vi "PH_Sequencer_Watch.panel.vi"() -> ()   [LabVIEW 2014, in "PH_Sequencer_Watch.lvlib"]
uses:
  PH_Sequencer_Watch.lvlib
  PH_Beamline_Chief/PH_Beamline_Chief.Section.ctl
  PH_Basics/PH_SystemInformation/PH_SystemInformation.GUI Refs.ctl
  PH_BeamlineInformation/PH_BeamlineInformation.Powermeter.ctl
  PH_BeamlineInformation/PH_BeamlineInformation.Efficiency.ctl
  PH_Basics/PH_PP_Common/PH_PP_Common.PUs.ctl
  PH_Sequencer_Watch.Head Information.ctl
  PH_BeamlineInformation/PH_BeamlineInformation.GUI Ref.ctl
  PH_Basics/PH_Common/PH_Common.lvlib
  PH_Beamline_Chief/PH_Beamline_Chief.lvlib
  PH_BeamlineInformation/PH_BeamlineInformation.lvlib
  PH_Basics/PH_PP_Common/PH_PP_Common.lvlib
  PH_Basics/PH_SystemInformation/PH_SystemInformation.lvlib
  PH_Basics/PH_Class/PH_Class.lvlib
panel:
  out "PA 45 DP Voltage":cluster{dbl, dbl}(slide)={99999.0, 0.0} scale=0.0..20.0
  out "PPPA 45mm DP":bool caption="45 DP"
  out "PA 45 Voltage":cluster{dbl, dbl}(slide)={99999.0, 0.0} scale=0.0..20.0
  out "PPPA_45mm_MAIN_PU":bool caption="45"
  out "PA 19-2 Voltage":cluster{dbl, dbl}(slide)={99999.0, 0.0} scale=0.0..20.0
  out "PPPA_19mm_2_PU":bool caption="19-2"
  out "PA 19-1 Voltage":cluster{dbl, dbl}(slide)={99999.0, 0.0} scale=0.0..20.0
  out "PPPA_19mm_1_PU":bool caption="State PU"
  out "Z6_COS_Powermeter_CurrentValue":dbl=-1.0 caption="mJ"
  out "Z6_IR_Powermeter_CurrentValue":dbl=-1.0 caption="J"
  out "Z6_green_Powermeter_CurrentValue":dbl=-1.0 caption="J"
  out "PHELIX_Beamline_MA_LB_BL_Status 2":u32(colorbox)
  out "Experiment_VacuumControl_Experiment":bool caption="V"
  out "PA-Backreflection-Meas":bool caption="B"
  out "fs_Synchrolock_Watch":bool caption="S"
  in  "T2-Unit-Dummy":string caption="s"
  out "PHELIX_Timing_T2":i16 caption="T2"
  out "PHELIX_Beamline_PA_before_Bypass_BL_Status":u32(colorbox)
  out "PHELIX_Beamline_PA_BL_Status":u32(colorbox)
  out "PHELIX_Beamline_LB_TB2_BL_Status":u32(colorbox)
  out "PHELIX_Beamline_Z6_BL_Status":u32(colorbox)
  out "PHELIX_Beamline_LL_BL_Status":u32(colorbox)
  out "PHELIX_Beamline_MA_Exit_BL_Status":u32(colorbox)
  out "PHELIX_Beamline_PA_Exit_BL_Status":u32(colorbox)
  out "PHELIX_Beamline_PA_Input_BL_Status":u32(colorbox)
  out "PHELIX_Beamline_PA_UnDelay_BL_Status":u32(colorbox)
  out "PHELIX_Beamline_fs_YLF_BL_Status":u32(colorbox)
  out "PHELIX_Beamline_YLF_BL_Status 2":u32(colorbox)
  out "PHELIX_Beamline_ns_BL_Status 2":u32(colorbox)
  out "PHELIX_Beamline_PA_Bypass_BL_Status 3":u32(colorbox)
  out "PHELIX_Beamline_PA_Bypass_BL_Status 2":u32(colorbox)
  out "PHELIX_Beamline_PA_Bypass_BL_Status 1":u32(colorbox)
  out "PHELIX_Beamline_PA_Delay_BL_Status 3":u32(colorbox)
  out "PHELIX_Beamline_PA_Delay_BL_Status 1":u32(colorbox)
  out "PHELIX_Beamline_PA_Delay_BL_Status 2":u32(colorbox)
  out "PHELIX_Beamline_MA_Z6_BL_Status":u32(colorbox)
  out "PA_Exit_Powermeter_CurrentValue":dbl=-1.0 caption="J"
  out "MAS_Powermeter_CurrentValue":dbl=-1.0 caption="J"
  out "PHELIX_Beamline_MA_LB_BL_Status 1":u32(colorbox)
  out "PHELIX_Beamline_MA_LB_BL_Status":u32(colorbox)
  out "PHELIX_Beamline_YLF_BL_Status 1":u32(colorbox)
  out "PHELIX_Beamline_fs_BL_Status":u32(colorbox)
  out "PHELIX_Beamline_ns_BL_Status 1":u32(colorbox)
  out "PHELIX_Beamline_PA_LL_BL_Status 2":u32(colorbox)
  out "PHELIX_Beamline_PA_LL_BL_Status 1":u32(colorbox)
  out "PHELIX_Beamline_PA_MA_BL_Status":u32(colorbox)
  out "Countdown_Remaining_Time":string caption="ing_Time"
  out "MA PU FR Voltage":cluster{dbl, dbl}(slide)={99999.0, 0.0} scale=0.0..20.0
  out "PPMA_FR":bool caption="State PU"
  out "MA PU 5 Voltage":cluster{dbl, dbl}(slide)={99999.0, 0.0} scale=0.0..20.0
  out "PPMA_PU5":bool caption="State PU"
  out "MA PU 4 Voltage":cluster{dbl, dbl}(slide)={99999.0, 0.0} scale=0.0..20.0
  out "PPMA_PU4":bool caption="State PU"
  out "MA PU 3 Voltage":cluster{dbl, dbl}(slide)={99999.0, 0.0} scale=0.0..20.0
  out "PPMA_PU3":bool caption="State PU"
  out "MA PU 2 Voltage":cluster{dbl, dbl}(slide)={99999.0, 0.0} scale=0.0..20.0
  out "PPMA_PU2":bool caption="State PU"
  out "MA PU 1 Voltage":cluster{dbl, dbl}(slide)={99999.0, 0.0} scale=0.0..20.0
  out "PPMA_PU1":bool caption="State PU"
  out "PHELIX_PSDB-Controller_Shot-ID":i32 caption="Shot ID"
  out "PHELIX_Sequencer_1":string="no info" caption="Sequencer State"
  out "PHELIX_Timing_Mode":enum32{"10 Hz", "0.5 Hz", "Shot"}(radio) caption="Modeselector"
  in  "Delete":bool
  out "PIL_Exp4_ShutterDisabled":u32(colorbox) caption="Z6 enabled"
  out "PIL_Exp1_ShutterDisabled":u32(colorbox) caption="Exp 1 enabled"
  out "PIL_Exp2_ShutterDisabled":u32(colorbox) caption="Exp 2 enabled"
  out "PIL_Exp3_ShutterDisabled":u32(colorbox) caption="Exp 3 enabled"
  out "PIL_disabled_mainamp":u32(colorbox) caption="MA enabled"
  out "PIL_NA_Chain":u32(colorbox) caption="Emergency off"
  out "PIL_disabled_laser":u32(colorbox) caption="Laser enabled"
  out "PIL_disabled_preamp":u32(colorbox) caption="PA enabled"
  out "error out":errorcluster
  in  "error in (no error)":errorcluster
  in  "object ref":refnum<vi>
  out "PHELIX_Beamline_LB_TB3_BL_Status":u32(colorbox)
  # "PCS"
  # "3.40"
  # "19 DP"
  # "Z6"
  # "MA"
  # "ns-FE"
  # "fs-FE"
  # "YLF"
  # "FR"
  # "5"
  # "4"
  # "3"
  # "2"
  # "1"
  # "Exp LB"
  # "LL"
  # "PA"
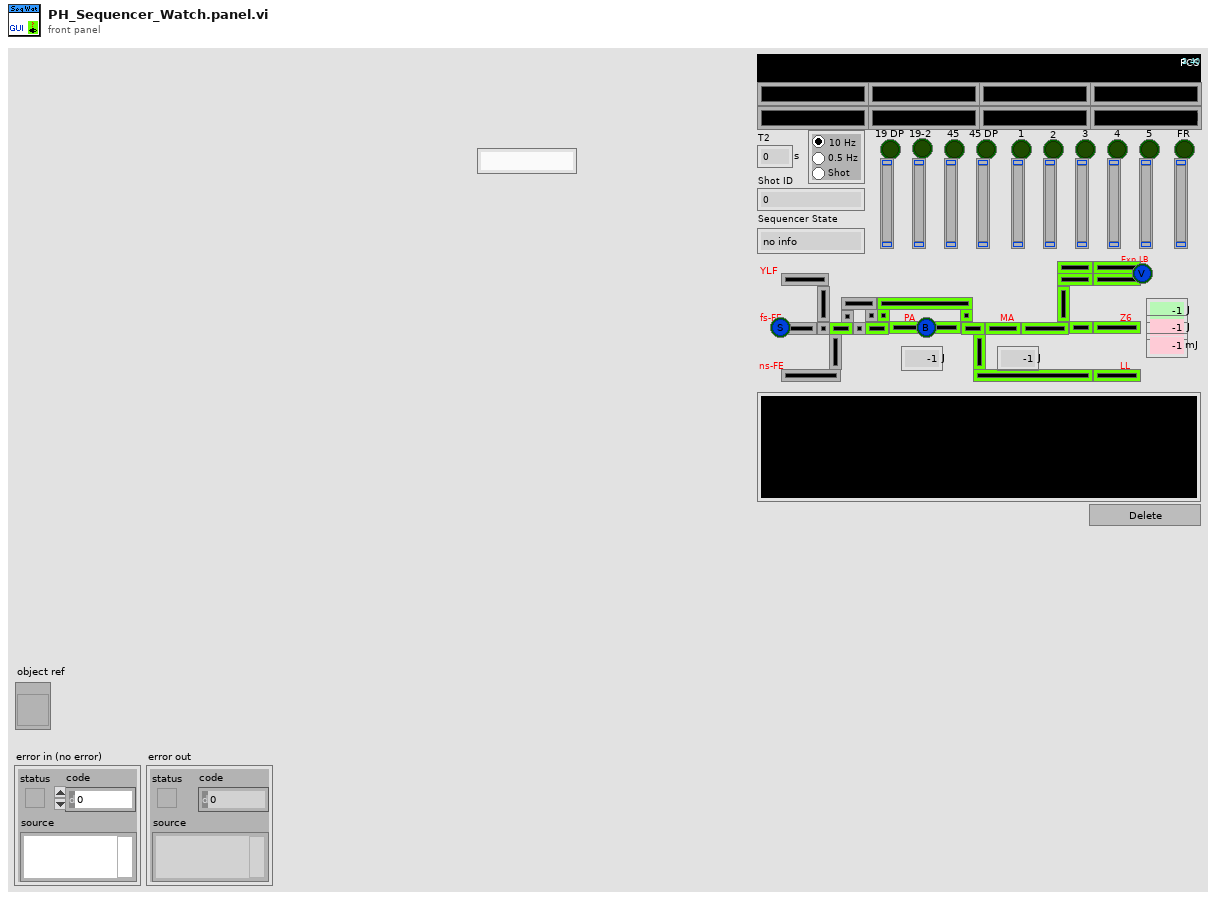
[diagram p1: front panel]
types:
  T1 = typedef "PH_BeamlineInformation.lvlib/PH_BeamlineInformation.GUI Ref.ctl" = cluster{"BL Elements":cluster{"GUI Ref":refnum<vi>, "Beamline Section":T2}[], "Powermeters":T3, "Efficiency GUI Refs":T4, "Head GUI Refs":cluster{"PA - 19 - 1":cluster{"in Use":refnum<vi>, "voltage":refnum<vi>}, "PA - 19 - 2":cluster{"in Use":refnum<vi>, "voltage":refnum<vi>}, "PA - 45":cluster{"in Use":refnum<vi>, "voltage":refnum<vi>}, "PA - 45 - DP":cluster{"in Use":refnum<vi>, "voltage":refnum<vi>}, "MA - 1":cluster{"in Use":refnum<vi>, "voltage":refnum<vi>}, "MA - 2":cluster{"in Use":refnum<vi>, "voltage":refnum<vi>}, "MA - 3":cluster{"in Use":refnum<vi>, "voltage":refnum<vi>}, "MA - 4":cluster{"in Use":refnum<vi>, "voltage":refnum<vi>}, "MA - 5":cluster{"in Use":refnum<vi>, "voltage":refnum<vi>}, "MA - FR":cluster{"in Use":refnum<vi>, "voltage":refnum<vi>}}, "System Information GUI Refs":T5}
  T2 = typedef "PH_Beamline_Chief.lvlib/PH_Beamline_Chief.Section.ctl" = enum16{"None", "YLF", "fs", "fs-YLF", "ns", "PA-Input", "PA-Undelay", "PA-Delay", "PA-before-Bypass", "PA", "PA-Bypass", "PA-Exit", "PA-LL", "LL", "PA-MA", "MA-Exit", "MA-Z6", "Z6", "MA-LB", "LB-TB2", "LB-TB3"}
  T3 = typedef "PH_BeamlineInformation.lvlib/PH_BeamlineInformation.Powermeter.ctl" = cluster{"ns FE":cluster{"GUI Ref":refnum<vi>, "Value":dbl}, "fs FE":cluster{"GUI Ref":refnum<vi>, "Value":dbl}, "PA":cluster{"GUI Ref":refnum<vi>, "Value":dbl}, "MA":cluster{"GUI Ref":refnum<vi>, "Value":dbl}, "Z6 green":cluster{"GUI Ref":refnum<vi>, "Value":dbl}, "Z6 IR":cluster{"GUI Ref":refnum<vi>, "Value":dbl}, "Z6 COS":cluster{"GUI Ref":refnum<vi>, "Value":dbl}}
  T4 = typedef "PH_BeamlineInformation.lvlib/PH_BeamlineInformation.Efficiency.ctl" = cluster{"PA Gain":cluster{"GUI Ref":refnum<vi>, "Value":dbl}, "MA Gain":cluster{"GUI Ref":refnum<vi>, "Value":dbl}, "Z6 green Conversion":cluster{"GUI Ref":refnum<vi>, "Value":dbl}, "Z6 Comp Losses":cluster{"GUI Ref":refnum<vi>, "Value":dbl}}
  T5 = typedef "PH_SystemInformation.lvlib/PH_SystemInformation.GUI Refs.ctl" = cluster{"Laser":refnum<vi>, "PreAmp":refnum<vi>, "MainAmp":refnum<vi>, "Emergency Off":refnum<vi>, "Exp 1":refnum<vi>, "Exp 2":refnum<vi>, "Exp 3":refnum<vi>, "Exp 4":refnum<vi>, "Timing Mode GUI Ref":refnum<vi>}
  T6 = typedef "PH_Sequencer_Watch.lvlib/PH_Sequencer_Watch.Head Information.ctl" = cluster{"Ref Volt":refnum<vi>, "PU":T7}
  T7 = typedef "PH_PP_Common.lvlib/PH_PP_Common.PUs.ctl" = enum16{"no Info", "PA-19mm-1", "PA-19mm-2", "PA-45mm-PILC", "PA-45mm-MAIN", "MA-PU-1", "MA-PU-2", "MA-PU-3", "MA-PU-4", "MA-PU-5", "MA-PU-6", "MA-FR", "MA-PILC", "PA-45mm-DP"}
  T8 = cluster{"PA - 19 - 1":cluster{"in Use":refnum<vi>, "voltage":refnum<vi>}, "PA - 19 - 2":cluster{"in Use":refnum<vi>, "voltage":refnum<vi>}, "PA - 45":cluster{"in Use":refnum<vi>, "voltage":refnum<vi>}, "PA - 45 - DP":cluster{"in Use":refnum<vi>, "voltage":refnum<vi>}, "MA - 1":cluster{"in Use":refnum<vi>, "voltage":refnum<vi>}, "MA - 2":cluster{"in Use":refnum<vi>, "voltage":refnum<vi>}, "MA - 3":cluster{"in Use":refnum<vi>, "voltage":refnum<vi>}, "MA - 4":cluster{"in Use":refnum<vi>, "voltage":refnum<vi>}, "MA - 5":cluster{"in Use":refnum<vi>, "voltage":refnum<vi>}, "MA - FR":cluster{"in Use":refnum<vi>, "voltage":refnum<vi>}}
  T9 = cluster{"GUI Ref":refnum<vi>, "Beamline Section":T2}
  T10 = typedef "PH_Sequencer_Watch.lvlib/PH_Sequencer_Watch.i attribute.ctl" = cluster{"GUI Refs":cluster{"Shot ID":refnum<vi>, "Sequencer SM State":refnum<vi>, "Remaining Time":refnum<vi>, "PHELIX_Timing_T2":refnum<vi>, "T2-Unit-Dummy":refnum<vi>, "fs_Synchrolock_Watch":refnum<vi>, "Experiment_Vacuum_Control_Experiment":refnum<vi>}, "Status Synchrolock":T11, "Exp - Pressure":dbl, "Exp - Limit":dbl, "Heads":T6[], "Refs BooleanState":refnum<vi>[]}
  T11 = typedef "PH_StatusHandler.lvlib/PH_StatusHandler.Status.ctl" = i16
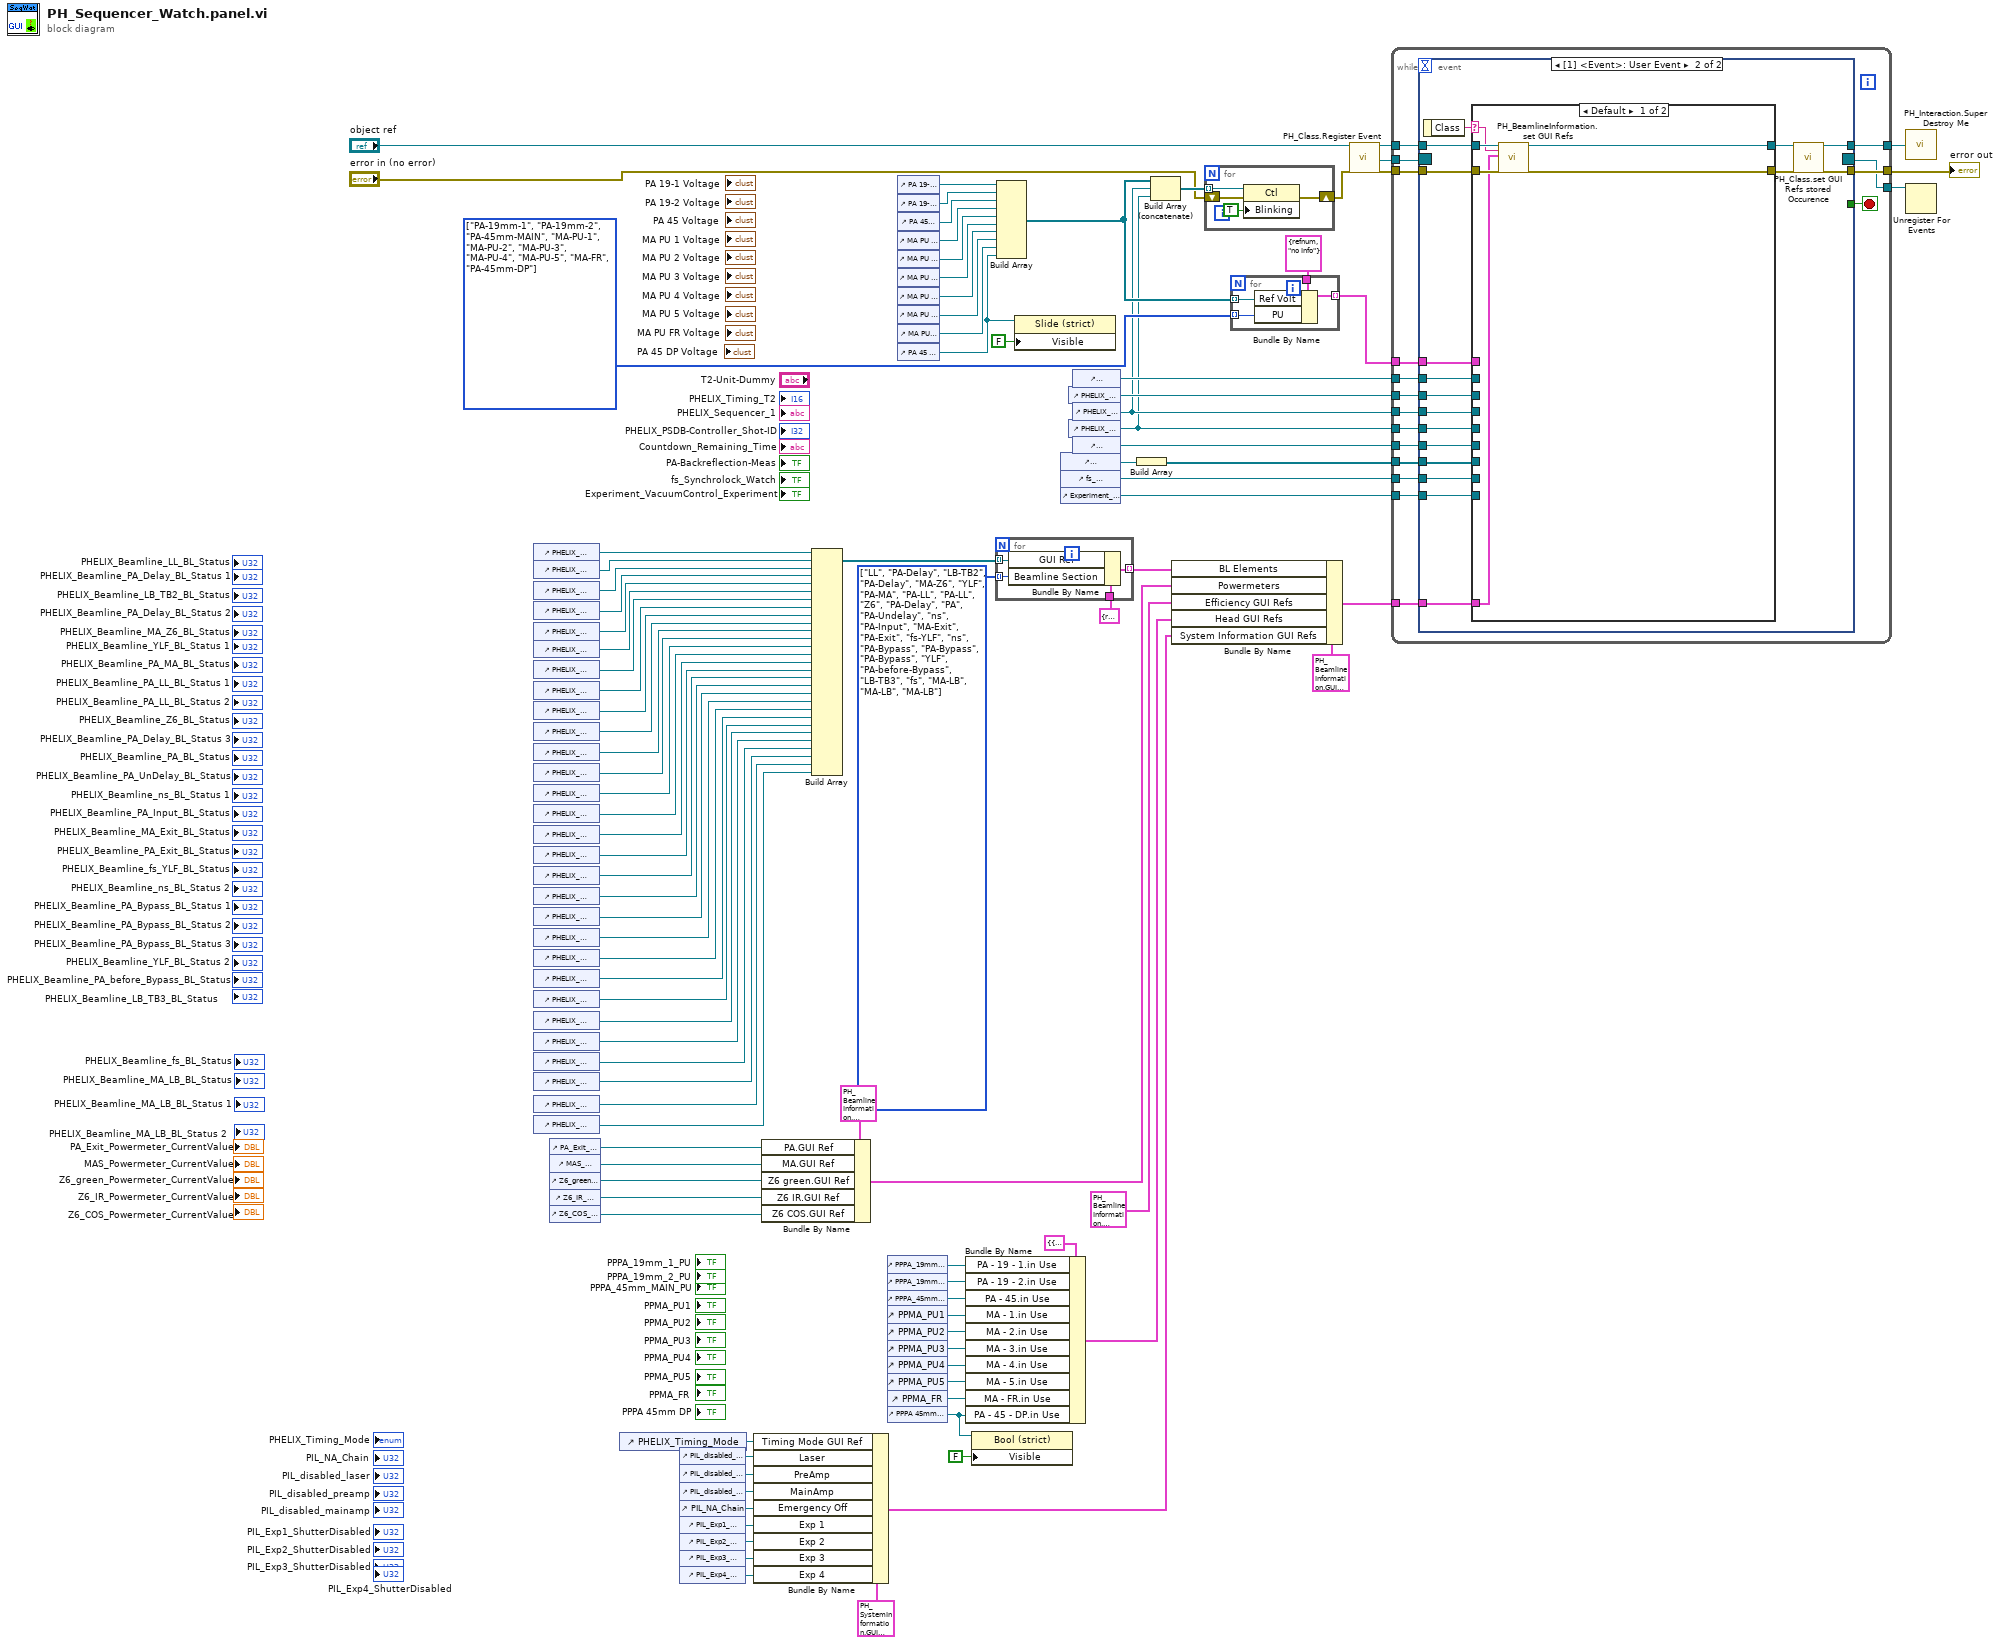
[diagram p0: block diagram]
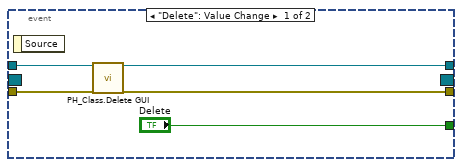
[diagram p2: hidden frame]
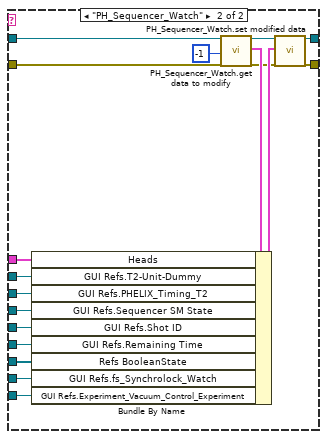
[diagram p3: hidden frame]
diagram:
  w25 = T7[] [enum."PA-19mm-1", enum."PA-19mm-2", enum."PA-45mm-MAIN", enum."MA-PU-1", enum."MA-PU-2", enum."MA-PU-3", enum."MA-PU-4", enum."MA-PU-5", enum."MA-FR", enum."PA-45mm-DP"] items=["no Info", "PA-19mm-1", "PA-19mm-2", "PA-45mm-PILC", "PA-45mm-MAIN", "MA-PU-1", "MA-PU-2", "MA-PU-3", "MA-PU-4", "MA-PU-5", "MA-PU-6", "MA-FR", "MA-PILC", "PA-45mm-DP"]
  w49 = T2[] [enum."LL", enum."PA-Delay", enum."LB-TB2", enum."PA-Delay", enum."MA-Z6", enum."YLF", enum."PA-MA", enum."PA-LL", enum."PA-LL", enum."Z6", enum."PA-Delay", enum."PA", enum."PA-Undelay", enum."ns", enum."PA-Input", enum."MA-Exit", enum."PA-Exit", enum."fs-YLF", enum."ns", enum."PA-Bypass", enum."PA-Bypass", enum."PA-Bypass", enum."YLF", enum."PA-before-Bypass", enum."LB-TB3", enum."fs", enum."MA-LB", enum."MA-LB", enum."MA-LB"] items=["None", "YLF", "fs", "fs-YLF", "ns", "PA-Input", "PA-Undelay", "PA-Delay", "PA-before-Bypass", "PA", "PA-Bypass", "PA-Exit", "PA-LL", "LL", "PA-MA", "MA-Exit", "MA-Z6", "Z6", "MA-LB", "LB-TB2", "LB-TB3"]
  n1 = control-ref of="PHELIX_Beamline_LL_BL_Status"() -> (w91:refnum<vi>)
  n2 = control-ref of="PHELIX_Beamline_PA_Delay_BL_Status 1"() -> (w90:refnum<vi>)
  n3 = control-ref of="PHELIX_Beamline_LB_TB2_BL_Status"() -> (w89:refnum<vi>)
  n4 = control-ref of="PHELIX_Beamline_PA_Delay_BL_Status 2"() -> (w88:refnum<vi>)
  n5 = control-ref of="PHELIX_Beamline_MA_Z6_BL_Status"() -> (w87:refnum<vi>)
  n6 = control-ref of="PHELIX_Beamline_YLF_BL_Status 1"() -> (w86:refnum<vi>)
  n7 = control-ref of="PHELIX_Beamline_PA_MA_BL_Status"() -> (w85:refnum<vi>)
  n8 = control-ref of="PHELIX_Beamline_PA_LL_BL_Status 1"() -> (w84:refnum<vi>)
  n9 = control-ref of="PHELIX_Beamline_PA_LL_BL_Status 2"() -> (w83:refnum<vi>)
  n10 = control-ref of="PHELIX_Beamline_Z6_BL_Status"() -> (w82:refnum<vi>)
  n11 = control-ref of="PHELIX_Beamline_PA_Delay_BL_Status 3"() -> (w81:refnum<vi>)
  n12 = control-ref of="PHELIX_Beamline_PA_BL_Status"() -> (w80:refnum<vi>)
  n13 = control-ref of="PHELIX_Beamline_PA_UnDelay_BL_Status"() -> (w79:refnum<vi>)
  n14 = control-ref of="PHELIX_Beamline_ns_BL_Status 1"() -> (w78:refnum<vi>)
  n15 = control-ref of="PHELIX_Beamline_PA_Input_BL_Status"() -> (w77:refnum<vi>)
  n16 = control-ref of="PHELIX_Beamline_MA_Exit_BL_Status"() -> (w76:refnum<vi>)
  n17 = control-ref of="PHELIX_Beamline_PA_Exit_BL_Status"() -> (w75:refnum<vi>)
  n18 = control-ref of="PHELIX_Beamline_fs_YLF_BL_Status"() -> (w74:refnum<vi>)
  n19 = control-ref of="PHELIX_Beamline_ns_BL_Status 2"() -> (w73:refnum<vi>)
  n20 = control-ref of="PHELIX_Beamline_PA_Bypass_BL_Status 1"() -> (w72:refnum<vi>)
  n21 = control-ref of="PHELIX_Beamline_PA_Bypass_BL_Status 2"() -> (w71:refnum<vi>)
  n22 = control-ref of="PHELIX_Beamline_PA_Bypass_BL_Status 3"() -> (w70:refnum<vi>)
  n23 = control-ref of="PHELIX_Beamline_YLF_BL_Status 2"() -> (w69:refnum<vi>)
  n24 = control-ref of="PHELIX_Beamline_PA_before_Bypass_BL_Status"() -> (w68:refnum<vi>)
  n25 = control-ref of="PHELIX_Beamline_LB_TB3_BL_Status"() -> (w56:refnum<vi>)
  n26 = control-ref of="PHELIX_Beamline_fs_BL_Status"() -> (w55:refnum<vi>)
  n27 = control-ref of="PHELIX_Beamline_MA_LB_BL_Status"() -> (w54:refnum<vi>)
  n28 = control-ref of="PHELIX_Beamline_MA_LB_BL_Status 1"() -> (w53:refnum<vi>)
  n29 = control-ref of="PHELIX_Beamline_MA_LB_BL_Status 2"() -> (w52:refnum<vi>)
  n30 = control-ref of="PA_Exit_Powermeter_CurrentValue"() -> (w47:refnum<vi>)
  n31 = control-ref of="MAS_Powermeter_CurrentValue"() -> (w46:refnum<vi>)
  n32 = control-ref of="Z6_green_Powermeter_CurrentValue"() -> (w45:refnum<vi>)
  n33 = control-ref of="Z6_IR_Powermeter_CurrentValue"() -> (w44:refnum<vi>)
  n34 = control-ref of="Z6_COS_Powermeter_CurrentValue"() -> (w43:refnum<vi>)
  n35 = control-ref of="PHELIX_Timing_Mode"() -> (w22:refnum<vi>)
  n36 = control-ref of="PIL_disabled_laser"() -> (w66:refnum<vi>)
  n37 = control-ref of="PIL_disabled_preamp"() -> (w65:refnum<vi>)
  n38 = control-ref of="PIL_disabled_mainamp"() -> (w64:refnum<vi>)
  n39 = control-ref of="PIL_NA_Chain"() -> (w63:refnum<vi>)
  n40 = control-ref of="PIL_Exp1_ShutterDisabled"() -> (w62:refnum<vi>)
  n41 = control-ref of="PIL_Exp2_ShutterDisabled"() -> (w61:refnum<vi>)
  n42 = control-ref of="PIL_Exp3_ShutterDisabled"() -> (w60:refnum<vi>)
  n43 = control-ref of="PIL_Exp4_ShutterDisabled"() -> (w59:refnum<vi>)
  n44 = Bundle By Name(cluster=T5 {"Laser"=refnum, "PreAmp"=refnum, "MainAmp"=refnum, "Emergency Off"=refnum, "Exp 1"=refnum, "Exp 2"=refnum, "Exp 3"=refnum, "Exp 4"=refnum, "Timing Mode GUI Ref"=refnum} ("7Color GUI Refs"), "Timing Mode GUI Ref"=w22, "Laser"=w66, "PreAmp"=w65, "MainAmp"=w64, "Emergency Off"=w63, "Exp 1"=w62, "Exp 2"=w61, "Exp 3"=w60, "Exp 4"=w59) -> (w17:T5)
  n45 = Bundle By Name(cluster=T3 {"ns FE"={"GUI Ref"=refnum, "Value"=-1.0}, "fs FE"={"GUI Ref"=refnum, "Value"=-1.0}, "PA"={"GUI Ref"=refnum, "Value"=-1.0}, "MA"={"GUI Ref"=refnum, "Value"=-1.0}, "Z6 green"={"GUI Ref"=refnum, "Value"=-1.0}, "Z6 IR"={"GUI Ref"=refnum, "Value"=-1.0}, "Z6 COS"={"GUI Ref"=refnum, "Value"=-1.0}} ("Powermeters"), "PA.GUI Ref"=w47, "MA.GUI Ref"=w46, "Z6 green.GUI Ref"=w45, "Z6 IR.GUI Ref"=w44, "Z6 COS.GUI Ref"=w43) -> (w19:T3)
  n46 = Build Array(w91, w90, w89, w88, w87, w86, w85, w84, w83, w82, w81, w80, w79, w78, w77, w76, w75, w74, w73, w72, w71, w70, w69, w68, w56, w55, w54, w53, w52) -> (w50:refnum<vi>[])
  n47 = control-ref of="PPPA_19mm_1_PU"() -> (w42:refnum<vi>)
  n48 = control-ref of="PPPA_19mm_2_PU"() -> (w41:refnum<vi>)
  n49 = control-ref of="PPPA_45mm_MAIN_PU"() -> (w40:refnum<vi>)
  n50 = control-ref of="PPMA_PU1"() -> (w39:refnum<vi>)
  n51 = control-ref of="PPMA_PU2"() -> (w38:refnum<vi>)
  n52 = control-ref of="PPMA_PU3"() -> (w37:refnum<vi>)
  n53 = control-ref of="PPMA_PU4"() -> (w36:refnum<vi>)
  n54 = control-ref of="PPMA_PU5"() -> (w35:refnum<vi>)
  n55 = control-ref of="PPMA_FR"() -> (w34:refnum<vi>)
  n56 = control-ref of="PPPA 45mm DP"() -> (w28:refnum<vi>)
  n57 = control-ref of="PA 19-1 Voltage"() -> (w101:refnum<vi>)
  n58 = control-ref of="PA 19-2 Voltage"() -> (w100:refnum<vi>)
  n59 = control-ref of="PA 45 Voltage"() -> (w94:refnum<vi>)
  n60 = control-ref of="MA PU 1 Voltage"() -> (w99:refnum<vi>)
  n61 = control-ref of="MA PU 2 Voltage"() -> (w98:refnum<vi>)
  n62 = control-ref of="MA PU 3 Voltage"() -> (w97:refnum<vi>)
  n63 = control-ref of="MA PU 4 Voltage"() -> (w96:refnum<vi>)
  n64 = control-ref of="MA PU 5 Voltage"() -> (w95:refnum<vi>)
  n65 = control-ref of="MA PU FR Voltage"() -> (w57:refnum<vi>)
  n66 = control-ref of="PA 45 DP Voltage"() -> (w30:refnum<vi>)
  n67 = Bundle By Name(cluster=T8 {"PA - 19 - 1"={"in Use"=refnum, "voltage"=refnum}, "PA - 19 - 2"={"in Use"=refnum, "voltage"=refnum}, "PA - 45"={"in Use"=refnum, "voltage"=refnum}, "PA - 45 - DP"={"in Use"=refnum, "voltage"=refnum}, "MA - 1"={"in Use"=refnum, "voltage"=refnum}, "MA - 2"={"in Use"=refnum, "voltage"=refnum}, "MA - 3"={"in Use"=refnum, "voltage"=refnum}, "MA - 4"={"in Use"=refnum, "voltage"=refnum}, "MA - 5"={"in Use"=refnum, "voltage"=refnum}, "MA - FR"={"in Use"=refnum, "voltage"=refnum}} ("Head GUI Refs"), "PA - 19 - 1.in Use"=w42, "PA - 19 - 2.in Use"=w41, "PA - 45.in Use"=w40, "MA - 1.in Use"=w39, "MA - 2.in Use"=w38, "MA - 3.in Use"=w37, "MA - 4.in Use"=w36, "MA - 5.in Use"=w35, "MA - FR.in Use"=w34, "PA - 45 - DP.in Use"=w28) -> (w1:T8)
  n68 = property class="Bool (strict)"(reference=w28, "Visible"=FALSE) -> ()  [unwired: 1 in, 2 out]
  n69 = for {
    tunnel: T9 {"GUI Ref"=refnum, "Beamline Section"=enum."None"} ("BL Element") -> [w105]
    tunnel: [w104] -> w20 mode=indexing
    tunnel: w50 -> [w103] mode=indexing
    tunnel: w49 -> [w102] mode=indexing
    n70 = Bundle By Name(cluster=w105, "GUI Ref"=w103, "Beamline Section"=w102) -> (w104:T9)
  }
  n71 = Build Array(w101, w100, w94, w99, w98, w97, w96, w95, w57, w30) -> (w31:refnum<vi>[])
  n72 = property class="Slide (strict)"(reference=w30, "Visible"=FALSE) -> ()  [unwired: 1 in, 2 out]
  n73 = control-ref of="PA-Backreflection-Meas"() -> (w58:refnum<vi>)
  n74 = control-ref of="fs_Synchrolock_Watch"() -> (w6:refnum<vi>)
  n75 = control-ref of="Experiment_VacuumControl_Experiment"() -> (w5:refnum<vi>)
  n76 = control-ref of="PHELIX_Timing_T2"() -> (w11:refnum<vi>)
  n77 = control-ref of="PHELIX_PSDB-Controller_Shot-ID"() -> (w9:refnum<vi>)
  n78 = control-ref of="T2-Unit-Dummy"() -> (w12:refnum<vi>)
  n79 = control-ref of="PHELIX_Sequencer_1"() -> (w10:refnum<vi>)
  n80 = control-ref of="Countdown_Remaining_Time"() -> (w8:refnum<vi>)
  n81 = Build Array(w58) -> (w7:refnum<vi>[])
  n82 = Build Array (concatenate)(w31, w10, w9) -> (w32:refnum<vi>[])
  n83 = Bundle By Name(cluster=T1 {"BL Elements"=[], "Powermeters"={"ns FE"={"GUI Ref"=refnum, "Value"=-1.0}, "fs FE"={"GUI Ref"=refnum, "Value"=-1.0}, "PA"={"GUI Ref"=refnum, "Value"=-1.0}, "MA"={"GUI Ref"=refnum, "Value"=-1.0}, "Z6 green"={"GUI Ref"=refnum, "Value"=-1.0}, "Z6 IR"={"GUI Ref"=refnum, "Value"=-1.0}, "Z6 COS"={"GUI Ref"=refnum, "Value"=-1.0}}, "Efficiency GUI Refs"={"PA Gain"={"GUI Ref"=refnum, "Value"=-1.0}, "MA Gain"={"GUI Ref"=refnum, "Value"=-1.0}, "Z6 green Conversion"={"GUI Ref"=refnum, "Value"=-1.0}, "Z6 Comp Losses"={"GUI Ref"=refnum, "Value"=-1.0}}, "Head GUI Refs"={"PA - 19 - 1"={"in Use"=refnum, "voltage"=refnum}, "PA - 19 - 2"={"in Use"=refnum, "voltage"=refnum}, "PA - 45"={"in Use"=refnum, "voltage"=refnum}, "PA - 45 - DP"={"in Use"=refnum, "voltage"=refnum}, "MA - 1"={"in Use"=refnum, "voltage"=refnum}, "MA - 2"={"in Use"=refnum, "voltage"=refnum}, "MA - 3"={"in Use"=refnum, "voltage"=refnum}, "MA - 4"={"in Use"=refnum, "voltage"=refnum}, "MA - 5"={"in Use"=refnum, "voltage"=refnum}, "MA - FR"={"in Use"=refnum, "voltage"=refnum}}, "System Information GUI Refs"={"Laser"=refnum, "PreAmp"=refnum, "MainAmp"=refnum, "Emergency Off"=refnum, "Exp 1"=refnum, "Exp 2"=refnum, "Exp 3"=refnum, "Exp 4"=refnum, "Timing Mode GUI Ref"=refnum}} ("BeamlineInformation GUI Refs"), "BL Elements"=w20, "Powermeters"=w19, "Efficiency GUI Refs"=T4 {"PA Gain"={"GUI Ref"=refnum, "Value"=-1.0}, "MA Gain"={"GUI Ref"=refnum, "Value"=-1.0}, "Z6 green Conversion"={"GUI Ref"=refnum, "Value"=-1.0}, "Z6 Comp Losses"={"GUI Ref"=refnum, "Value"=-1.0}}, "Head GUI Refs"=w1, "System Information GUI Refs"=w17) -> (w15:T1)
  n84 = for {
    tunnel: w32 -> [w109] mode=indexing
    shift-right: [w108] -> w14
    shift-left: "error in (no error)" -> [w107]
    n85 = property class="Ctl"(reference=w109, error in=w107, "Blinking"=TRUE) -> (error out=w108:errorcluster)  [unwired: 1 out]
  }
  n86 = for {
    tunnel: w25 -> [w110] mode=indexing
    tunnel: w31 -> [w113] mode=indexing
    tunnel: T6 {"Ref Volt"=refnum, "PU"=enum."no Info"} ("Head Information") -> [w112]
    tunnel: [w111] -> w4 mode=indexing
    n87 = Bundle By Name(cluster=w112, "Ref Volt"=w113, "PU"=w110) -> (w111:T6)
  }
  n88 = call "PH_Class.Register Event.vi"("i ref in"="object ref", "error in (no error)"=w14) -> ("i ref out"=w24:refnum<vi>, "Event Registration Refnum"=w16:refnum<event-registration>, "error out"=w23:errorcluster)  [unwired: 15 in]
  n89 = while {
    tunnel: w24 -> [w127]
    tunnel: [w126] -> w93
    tunnel: [w129] -> w92
    tunnel: w23 -> [w128]
    tunnel: w16 -> [w125]
    tunnel: w15 -> [w124]
    tunnel: [w123] -> w13
    tunnel: w12 -> [w122]
    tunnel: w11 -> [w121]
    tunnel: w10 -> [w120]
    tunnel: w9 -> [w119]
    tunnel: w8 -> [w118]
    tunnel: w7 -> [w117]
    tunnel: w6 -> [w116]
    tunnel: w5 -> [w115]
    tunnel: w4 -> [w114]
    stop <- w130 stop-if-true
    n90 = event shown="[1] <Event>: User Event" {
      selector: w125 -> [_ _]
      dyn-events: [_ _] -> w123
      timeout: _ -> [_ _]
      tunnel: ["Delete" _] -> w130
      tunnel: w127 -> [w133 w152]
      tunnel: [w131 w138] -> w129
      tunnel: w128 -> [w134 w151]
      tunnel: [w132 w136] -> w126
      tunnel: w124 -> [_ w148]
      tunnel: w122 -> [_ w147]
      tunnel: w121 -> [_ w146]
      tunnel: w120 -> [_ w145]
      tunnel: w119 -> [_ w144]
      tunnel: w118 -> [_ w143]
      tunnel: w117 -> [_ w142]
      tunnel: w116 -> [_ w141]
      tunnel: w115 -> [_ w140]
      tunnel: w114 -> [_ w139]
      event "Delete": Value Change {
        n91 = event-data() -> ()  [unwired: 1 in, 1 out]
        n92 = call "PH_Class.Delete GUI.vi"("VI in"=w133, "error in (no error)"=w134) -> ("VI out"=w132:refnum<vi>, "error out"=w131:errorcluster)  [unwired: 16 in]
      }
      event User Event {
        n93 = event-data() -> ("Class"=w149:string)  [unwired: 1 in]
        n94 = case shown="Default" w149 {
          selector: w149 -> [w154 _]
          tunnel: w152 -> [w158 w171]
          tunnel: w151 -> [w157 w170]
          tunnel: [w156 w160] -> w137
          tunnel: [w155 w159] -> w150
          tunnel: w148 -> [w153 _]
          tunnel: w147 -> [_ w169]
          tunnel: w146 -> [_ w168]
          tunnel: w145 -> [_ w167]
          tunnel: w144 -> [_ w166]
          tunnel: w143 -> [_ w165]
          tunnel: w142 -> [_ w164]
          tunnel: w141 -> [_ w163]
          tunnel: w140 -> [_ w162]
          tunnel: w139 -> [_ w161]
          frame Default {
            n95 = call "PH_BeamlineInformation.set GUI Refs.vi"("Ref in"=w158, "Class"=w154, "BeamlineInformation GUI Refs"=w153, "error in"=w157) -> ("Ref out"=w156:refnum<vi>, "error out"=w155:errorcluster)  [unwired: 14 in]
          }
          frame "PH_Sequencer_Watch" {
            n96 = call "PH_Sequencer_Watch.get data to modify.vi"("i ref in"=w171, "ms timeout (10000)"=-1, "error in (no error)"=w170) -> ("i ref out"=w175:refnum<vi>, "i attribute"=w173:T10, "error out"=w172:errorcluster)  [unwired: 13 in, 1 out]
            n97 = Bundle By Name(cluster=w173, "Heads"=w161, "GUI Refs.T2-Unit-Dummy"=w169, "GUI Refs.PHELIX_Timing_T2"=w168, "GUI Refs.Sequencer SM State"=w167, "GUI Refs.Shot ID"=w166, "GUI Refs.Remaining Time"=w165, "Refs BooleanState"=w164, "GUI Refs.fs_Synchrolock_Watch"=w163, "GUI Refs.Experiment_Vacuum_Control_Experiment"=w162) -> (w174:T10)
            n98 = call "PH_Sequencer_Watch.set modified data.vi"("i ref in"=w175, "i attribute"=w174, "error in (no error)"=w172) -> ("i ref out"=w160:refnum<vi>, "error out"=w159:errorcluster)  [unwired: 15 in]
          }
        }
        n99 = call "PH_Class.set GUI Refs stored Occurence.vi"("i ref in"=w137, "error in (no error)"=w150) -> ("i ref out"=w136:refnum<vi>, "error out"=w138:errorcluster)  [unwired: 16 in]
      }
    }
  }
  "error out" <- w92
  n100 = call "PH_Interaction.Super Destroy Me.vi"("i ref out"=w93) -> ()
  n101 = Unregister For Events(event registration refnum=w13) -> ()  [unwired: 1 in, 1 out]
